vi "SUB_SORT_2D_ARRAY.vi"(8 "Index sort by":i32, 11 "array":string[][](array[string])) -> (3 "Sorted array":string[][](array[string]))   [LabVIEW 2015]
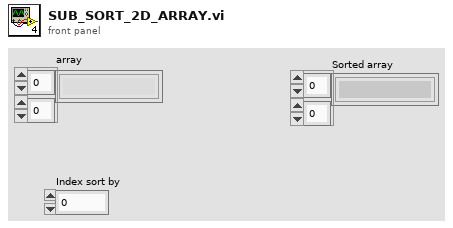
[diagram p1: front panel]
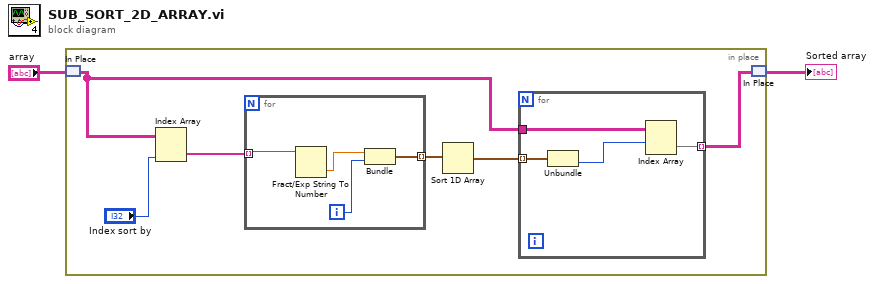
[diagram p0: block diagram]
diagram:
  n1 = in-place {
    n2 = in-place-match #1("array") -> (w4:string[][])
    n3 = Index Array(array=w4, index (col)="Index sort by") -> (element=w7:string[])  [unwired: 1 in]
    n4 = for {
      tunnel: w7 -> [w14] mode=indexing
      tunnel: [w15] -> w6 mode=indexing
      i -> [w16]
      n5 = Fract/Exp String To Number(string=w14) -> (number=w13:dbl)  [unwired: 3 in, 1 out]
      n6 = Bundle(w13, w16) -> (w15:cluster{dbl, i32})  [unwired: 1 in]
    }
    n7 = Sort 1D Array(array=w6) -> (sorted array=w5:cluster{dbl, i32}[])
    n8 = for {
      tunnel: w5 -> [w12] mode=indexing
      tunnel: w4 -> [w11]
      tunnel: [w9] -> w3 mode=indexing
      n9 = Unbundle(w12) -> (w10:i32)  [unwired: 1 out]
      n10 = Index Array(array=w11, index (row)=w10) -> (element=w9:string[])  [unwired: 1 in]
    }
    n11 = in-place-match #1(w3) -> (→"Sorted array":string[][])
  }
